vi "Schließen.vi"(8 "Error In":errorcluster caption="Fehler (Eingang)", 11 "Verbindungs-ID":refnum<k16>) -> (0 "Error Out":errorcluster caption="Fehler (Ausgang)")   [LabVIEW 2019, in "Thermostat Treiber.lvlib"]
uses:
  Thermostat Treiber.lvlib
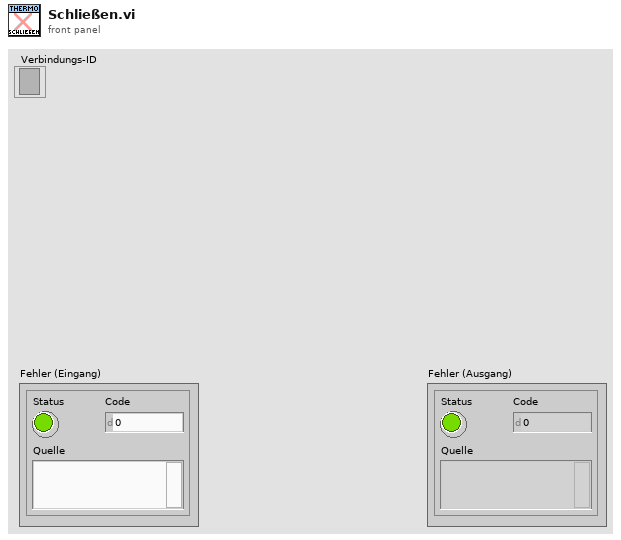
[diagram p1: front panel]
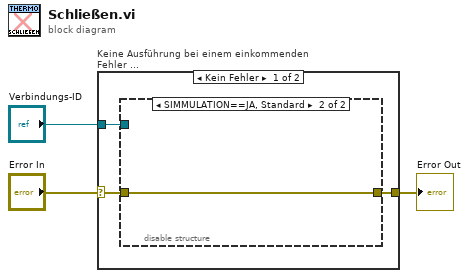
[diagram p0: block diagram]
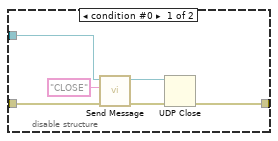
[diagram p2: hidden frame]
diagram:
  n1 = case "Keine Ausführung bei einem einkommenden Fehler ..." shown="Kein Fehler" "Error In" {
    selector: "Error In" -> [w5 w14]
    tunnel: [w6 w14] -> w2
    tunnel: "Verbindungs-ID" -> [w4 _]
    frame No Error {
      n2 = disable-structure shown="SIMMULATION==JA, Standard" {
        disable-tunnel: [w12 w13] -> w6
        disable-tunnel: w5 -> [w11 w13]
        disable-tunnel: w4 -> [w10 _]
        frame condition #0 {
          n3 = call "Send Message.vi"("Error In"=w11, "Nachricht"="CLOSE", "Verbindungs-ID in"=w10) -> ("Error Out"=w8:errorcluster, "Verbindungs-ID out"=w9:refnum<k16>)  [unwired: 7 in]
          n4 = UDP Close(connection ID=w9, 8:w8) -> (error out=w12:errorcluster)  [unwired: 1 out]
        }
        frame condition #1 (active) {
        }
      }
    }
    frame Error {
    }
  }
  "Error Out" <- w2
